vi "Main - Init Close Variable.vi"(6 "State":enum16{"Init", "Close"}(ring)=enum."Close", 8 "Error In":errorcluster) -> (0 "Error Out":errorcluster)   [LabVIEW 2020]
uses:
  Control/State - eFGV.ctl
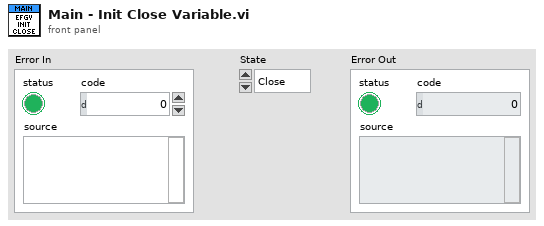
[diagram p1: front panel]
types:
  T1 = typedef "State - eFGV.ctl" = enum16{"Init", "Read", "Write", "Exit"}
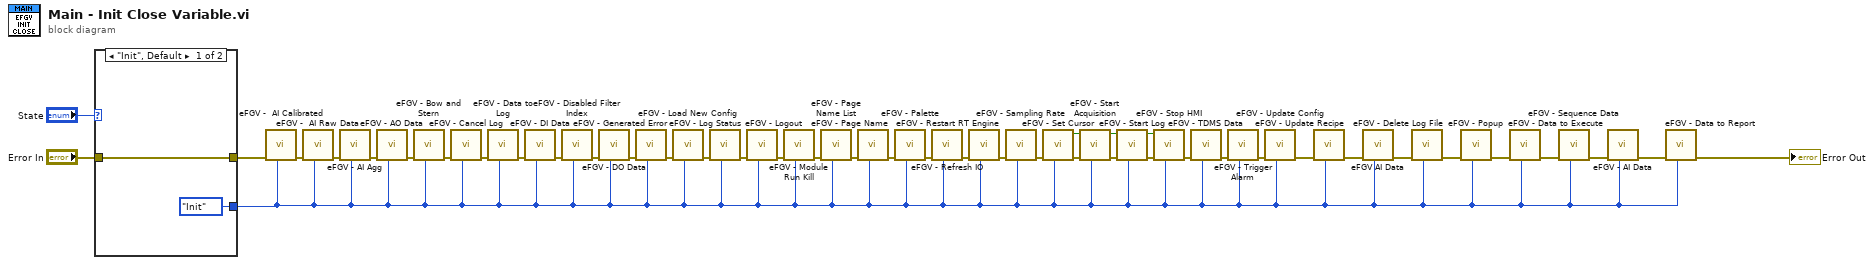
[diagram p0: block diagram]
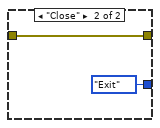
[diagram p2: hidden frame]
diagram:
  n1 = case shown="\"Init\", Default" "State" {
    tunnel: [State_-_eFGV."Init" ("Action") State_-_eFGV."Exit" ("Action")] -> w1
    tunnel: [w45 w47] -> w41
    tunnel: "Error In" -> [w45 w47]
    frame "Init", Default {
    }
    frame "Close" {
    }
  }
  n2 = call "eFGV -  AI Calibrated.vi"("States"=w1, "Error In"=w41) -> ("Error Out"=w40:errorcluster)  [unwired: 8 in, 1 out]
  n3 = call "eFGV -  AI Raw Data.vi"("States"=w1, "Error In"=w40) -> ("Error Out"=w39:errorcluster)  [unwired: 8 in, 1 out]
  n4 = call "eFGV - AI Agg.vi"("States"=w1, "Error In"=w39) -> ("Error Out"=w38:errorcluster)  [unwired: 8 in, 1 out]
  n5 = call "eFGV - AO Data.vi"("States"=w1, "Error In"=w38) -> ("Error Out"=w37:errorcluster)  [unwired: 8 in, 1 out]
  n6 = call "eFGV - Bow and Stern.vi"("Action"=w1, "Error In"=w37) -> ("Error Out"=w36:errorcluster)  [unwired: 7 in, 2 out]
  n7 = call "eFGV - Cancel Log.vi"("Action"=w1, "Error In"=w36) -> ("Error Out"=w35:errorcluster)  [unwired: 7 in, 2 out]
  n8 = call "eFGV - Data to Log.vi"("States"=w1, "Error In"=w35) -> ("Error Out"=w34:errorcluster)  [unwired: 8 in, 1 out]
  n9 = call "eFGV - DI Data.vi"("States"=w1, "Error In"=w34) -> ("Error Out"=w33:errorcluster)  [unwired: 7 in, 2 out]
  n10 = call "eFGV - Disabled Filter Index.vi"("eFGV States"=w1, "Error In"=w33) -> ("Error Out"=w32:errorcluster)  [unwired: 8 in, 1 out]
  n11 = call "eFGV - DO Data.vi"("States"=w1, "Error In"=w32) -> ("Error Out"=w31:errorcluster)  [unwired: 8 in, 1 out]
  n12 = call "eFGV - Generated Error.vi"("eFGV States"=w1, "Error In"=w31) -> ("Error Out"=w30:errorcluster)  [unwired: 8 in, 1 out]
  n13 = call "eFGV - Load New Config.vi"("eFGV States"=w1, "Error In"=w30) -> ("Error Out"=w29:errorcluster)  [unwired: 8 in, 1 out]
  n14 = call "eFGV - Log Status.vi"("States"=w1, "Error In"=w29) -> ("Error Out"=w28:errorcluster)  [unwired: 8 in, 1 out]
  n15 = call "eFGV - Logout.vi"("Action"=w1, "Error In"=w28) -> ("Error Out"=w27:errorcluster)  [unwired: 7 in, 2 out]
  n16 = call "eFGV - Module Run Kill.vi"("Action"=w1, "Error In"=w27) -> ("Error Out"=w26:errorcluster)  [unwired: 7 in, 2 out]
  n17 = call "eFGV - Page Name List.vi"("Action"=w1, "Error In"=w26) -> ("Error Out"=w25:errorcluster)  [unwired: 7 in, 2 out]
  n18 = call "eFGV - Page Name.vi"("Action"=w1, "Error In"=w25) -> ("Error Out"=w24:errorcluster)  [unwired: 7 in, 2 out]
  n19 = call "eFGV - Palette.vi"("eFGV States"=w1, "Error In"=w24) -> ("Error Out"=w23:errorcluster)  [unwired: 8 in, 1 out]
  n20 = call "eFGV - Refresh IO.vi"("States"=w1, "Error In"=w23) -> ("Error Out"=w22:errorcluster)  [unwired: 8 in, 1 out]
  n21 = call "eFGV - Restart RT Engine.vi"("Action"=w1, "Error In"=w22) -> ("Error Out"=w21:errorcluster)  [unwired: 7 in, 2 out]
  n22 = call "eFGV - Sampling Rate.vi"("eFGV States"=w1, "Error In"=w21) -> ("Error Out"=w20:errorcluster)  [unwired: 7 in, 2 out]
  n23 = call "eFGV - Set Cursor.vi"("FGV State"=w1, "Error In"=w20) -> ("Error Out"=w18:errorcluster, "Cursor Busy?"=w19:bool)  [unwired: 7 in, 1 out]
  n24 = call "eFGV - Start Acquisition.vi"("FGV State"=w1, "Error In"=w18, "Start Test"=w19) -> ("Error Out"=w16:errorcluster, "Start Out"=w17:bool)  [unwired: 6 in, 1 out]
  n25 = call "eFGV - Start Log.vi"("Action"=w1, "Error In"=w16, "Start Log"=w17) -> ("Error Out"=w14:errorcluster, "Start Log Out"=w15:bool)  [unwired: 6 in, 1 out]
  n26 = call "eFGV - Stop HMI.vi"("Action"=w1, "Error In"=w14, "Stop HMI? In"=w15) -> ("Error Out"=w9:errorcluster)  [unwired: 6 in, 2 out]
  n27 = call "eFGV - TDMS Data.vi"("Action"=w1, "Error In"=w9) -> ("Error Out"=w13:errorcluster)  [unwired: 7 in, 2 out]
  n28 = call "eFGV - Trigger Alarm.vi"("States"=w1, "Error In"=w13) -> ("Error Out"=w12:errorcluster)  [unwired: 8 in, 1 out]
  n29 = call "eFGV - Update Config.vi"("Action"=w1, "Error In"=w12) -> ("Error Out"=w11:errorcluster)  [unwired: 7 in, 2 out]
  n30 = call "eFGV - Update Recipe.vi"("FGV State"=w1, "Error In"=w11) -> ("Error Out"=w10:errorcluster)  [unwired: 7 in, 2 out]
  n31 = call "eFGV AI Data.vi"("States"=w1, "Error In"=w10) -> ("Error Out"=w8:errorcluster)  [unwired: 8 in, 1 out]
  n32 = call "eFGV - Delete Log File.vi"("Action"=w1, "Error In"=w8) -> ("Error Out"=w7:errorcluster)  [unwired: 7 in, 2 out]
  n33 = call "eFGV - Popup.vi"("Action"=w1, "Error In"=w7) -> ("Error Out"=w4:errorcluster)  [unwired: 7 in, 2 out]
  n34 = call "eFGV - Data to Execute.vi"("Action"=w1, "Error In"=w4) -> ("Error Out"=w5:errorcluster)  [unwired: 8 in, 1 out]
  n35 = call "eFGV - Sequence Data.vi"("States"=w1, "Error In"=w5) -> ("Error Out"=w6:errorcluster)  [unwired: 7 in, 2 out]
  n36 = call "eFGV - AI Data.vi"("States"=w1, "Error In"=w6) -> ("Error Out"=w3:errorcluster)  [unwired: 8 in, 1 out]
  n37 = call "eFGV - Data to Report.vi"("Action"=w1, "Error In"=w3) -> ("Error Out"=→"Error Out":errorcluster)  [unwired: 8 in, 1 out]
